vi "Actor Core.vi"(8 "error in":errorcluster, 11 "Controller in":refnum<class "Error Handler.lvclass">) -> (0 "error out":errorcluster, 3 "Actor out":refnum<class "Actor.lvclass">)   [LabVIEW 2017, in "Error Handler.lvlib" / "Error Handler.lvclass"]
doc: "(<B>Filename</B>: Actor Framework.lvlib:Actor.lvclass:Actor Core.vi)\n\nReceives messages to the actor, reacts to them, and initiates any error handling that may shut the actor down.\n\nDescendant classes may override this VI to append parallel tasks for the actor to complete while it handles messages. Overrides use the Call Parent Method node."
uses:
  Error Handler.lvclass
  <vilib>/ActorFramework/Actor/Actor.lvclass
  Game Engine/Game Engine/Game Engine.lvclass
  C:/Program Files (x86)/National Instruments/LabVIEW 2017/vi.lib/ActorFramework/Actor/Actor.lvclass
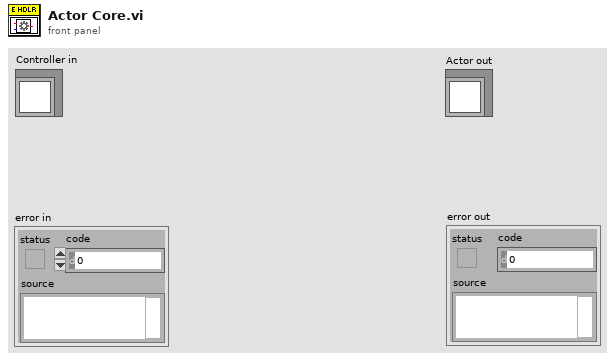
[diagram p1: front panel]
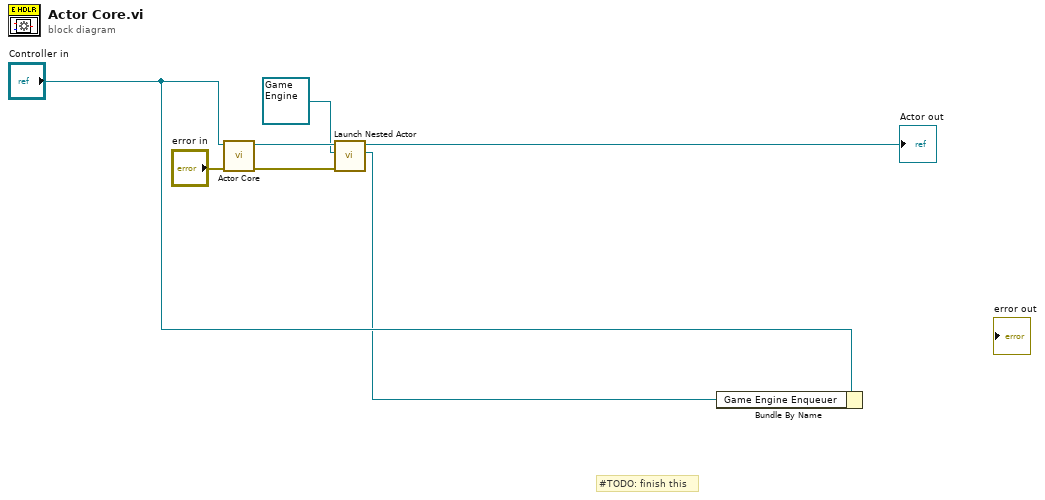
[diagram p0: block diagram]
diagram:
  # "#TODO: finish this"
  n1 = call-parent "Actor Core.vi"("error in"="error in", "Actor in"="Controller in") -> ("error out"=w5:errorcluster, "Actor out"=w6:refnum<class "Actor.lvclass">)  [unwired: 8 in]
  n2 = call <vilib>:"Launch Nested Actor.vi"("error in (no error)"=w5, "Nested Actor"=refnum<class "Game Engine.lvclass"> refnum ("Game Engine.lvlib:Game Engine.lvclass"), "Caller Actor in"=w6) -> ("Nested Actor's Enqueuer"=w3:refnum<class "Message Enqueuer.lvclass">, "Caller Actor out"=→"Actor out":refnum<class "Actor.lvclass">)  [unwired: 6 in, 1 out]
  n3 = Bundle By Name(cluster="Controller in", "Game Engine Enqueuer"=w3) -> ()  [unwired: 1 out]
